vi "servo-52.vi"(8 "error in (no error)":errorcluster, 11 "Enum":T1) -> (0 "error out":errorcluster)   [LabVIEW 2019]
uses:
  servo state.ctl
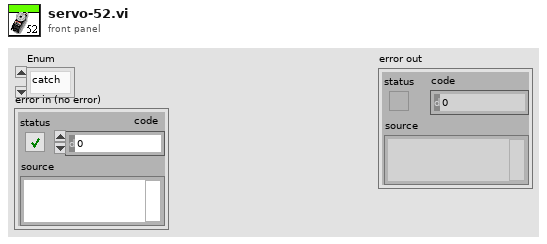
[diagram p1: front panel]
types:
  T1 = typedef "servo state.ctl" = enum16{"catch", "cam-1", "put", "side", "center", "side-2", "put-2"}
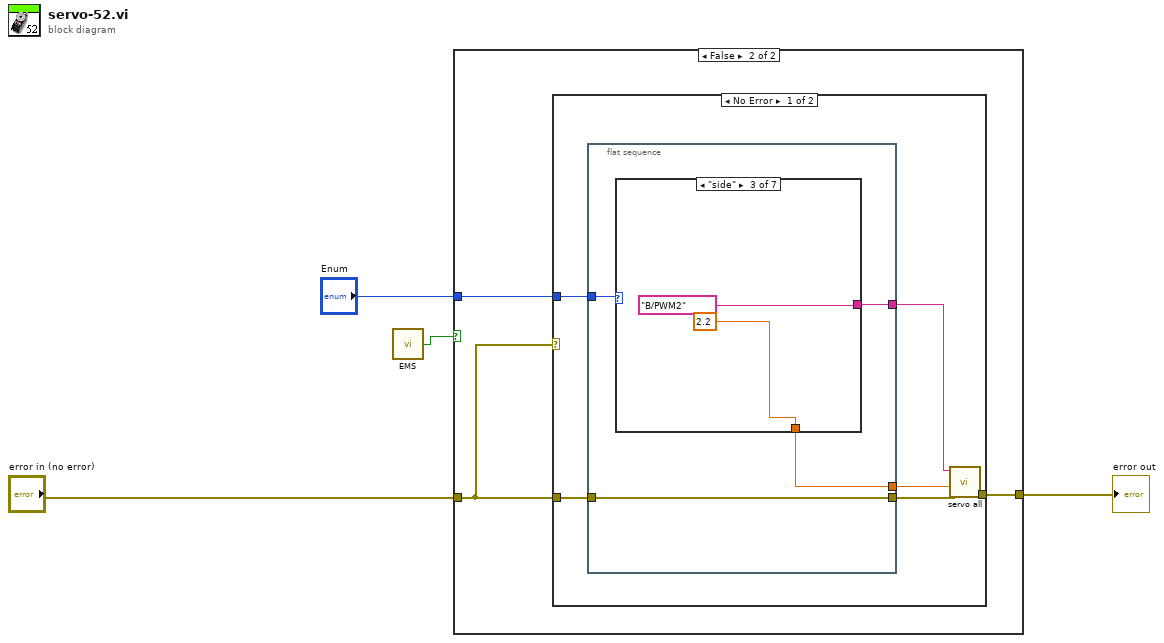
[diagram p0: block diagram]
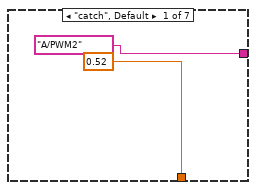
[diagram p3: hidden frame]
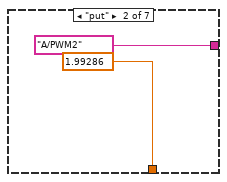
[diagram p4: hidden frame]
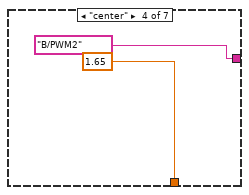
[diagram p5: hidden frame]
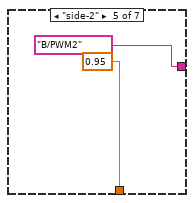
[diagram p6: hidden frame]
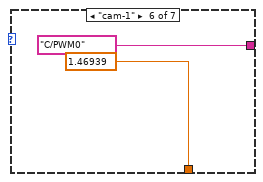
[diagram p7: hidden frame]
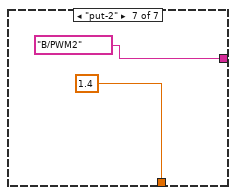
[diagram p8: hidden frame]
diagram:
  n1 = call "EMS.vi"() -> ("A/DIO4 (Pin 19)"=w1:bool)
  n2 = case shown="False" w1 {
    tunnel: "Enum" -> [_ w8]
    tunnel: [w5 w7] -> w3
    tunnel: "error in (no error)" -> [w5 w6]
    frame True {
    }
    frame False {
      n3 = case shown="No Error" w6 {
        tunnel: w8 -> [w14 _]
        tunnel: [w11 w33] -> w7
        tunnel: w6 -> [w9 w33]
        frame No Error {
          n4 = flat-sequence {
            tunnel: w14 -> [w18]
            tunnel: [w17] -> w13
            tunnel: [w16] -> w12
            tunnel: [w15] -> w10
            tunnel: w9 -> [w15]
            frame #0 {
              n5 = case shown="\"side\"" w18 {
                tunnel: [0.52 ("Numeric") 1.99286 ("Numeric") 2.2 ("Numeric") 1.65 ("Numeric") 0.95 ("Numeric") 1.46939 ("Numeric") 1.4 ("Numeric")] -> w17
                tunnel: [tag "A/PWM2" ("Channel Name") tag "A/PWM2" ("Channel Name") tag "B/PWM2" ("Channel Name") tag "B/PWM2" ("Channel Name") tag "B/PWM2" ("Channel Name") tag "C/PWM0" ("Channel Name") tag "B/PWM2" ("Channel Name")] -> w16
                frame "catch", Default {
                }
                frame "put" {
                }
                frame "side" {
                }
                frame "center" {
                }
                frame "side-2" {
                }
                frame "cam-1" {
                }
                frame "put-2" {
                }
              }
            }
          }
          n6 = call "servo all.vi"("error in (no error)"=w10, "Numeric"=w13, "Channel Name"=w12) -> ("error out"=w11:errorcluster)  [unwired: 8 in]
        }
        frame Error {
        }
      }
    }
  }
  "error out" <- w3
